vi "Wait For Current Play To Finish Core.vi"(9 "Timeout (seconds) (Infinity)":dbl, 11 "Sound Card in":refnum<class "Sound Card.lvclass">) -> (0 "error out":errorcluster, 3 "Sound Card out":refnum<class "Sound Card.lvclass">)   [LabVIEW 2017, in "Sound Card.lvclass"]
doc: "Wait for the sound currently playing on the player to complete. The default time out is \"Infinity\". Wiring a negative value will return an error."
uses:
  Sound Card.lvclass
  Sound Card.lvclass/Sound Card.ctl
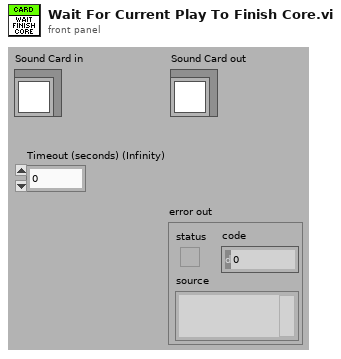
[diagram p1: front panel]
types:
  T1 = typedef "Sound Output Task ID.ctl" = u32
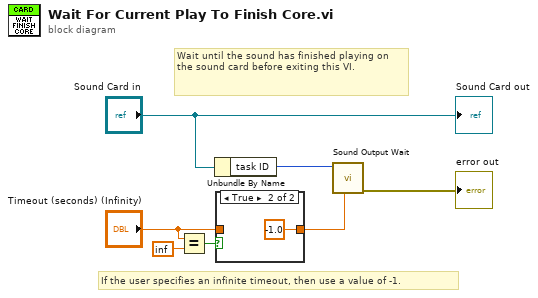
[diagram p0: block diagram]
diagram:
  # "If the user specifies an infinite timeout, then use a value of -1."
  # "Wait until the sound has finished playing on the sound card before exiting this VI."
  n1 = Equal?(x="Timeout (seconds) (Infinity)", y=inf) -> (x = y?=w5:bool)
  n2 = Unbundle By Name("Sound Card in") -> ("task ID"=w3:T1)
  n3 = case shown="True" w5 {
    tunnel: "Timeout (seconds) (Infinity)" -> [w8 _]
    tunnel: [w8 -1.0 ("Timeout (seconds) (Infinity)")] -> w1
    frame False {
    }
    frame True {
    }
  }
  n4 = call <vilib>:"Sound Output Wait.vi"("timeout (sec)"=w1, "task ID"=w3) -> ("error out"=→"error out":errorcluster)  [unwired: 8 in, 1 out]
  "Sound Card out" <- "Sound Card in"
